vi "LEBITplc.CreateScaleAndOffsetArray.vi"(2 "DBArray":string[][](array[string]), 3 "Info Array from DB":string[][](array[string])) -> (1 "Scale And Offset Array":string[][](array[string]))   [LabVIEW 2014, in "LEBITplc.lvlib"]
uses:
  LEBITplc.lvlib
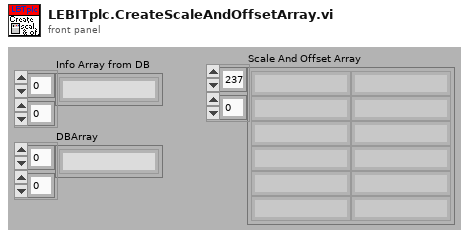
[diagram p1: front panel]
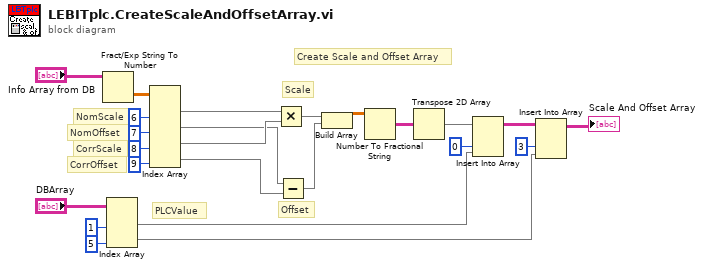
[diagram p0: block diagram]
diagram:
  # "Offset"
  # "Scale"
  # "PLCValue"
  # "Create Scale and Offset Array"
  # "CorrOffset"
  # "CorrScale"
  # "NomOffset"
  # "NomScale"
  n1 = Fract/Exp String To Number(string="Info Array from DB") -> (number=w24:dbl[][])  [unwired: 3 in, 1 out]
  n2 = Index Array(array="DBArray", index (col) #1=1 ("disabled index (col)"), index (col) #2=5 ("index (col)")) -> (element #1=w7:string[], element #2=w3:string[])  [unwired: 2 in]
  n3 = Index Array(array=w24, index (col) #1=6 ("index (col)"), index (col) #2=7 ("index (col)"), index (col) #3=8 ("index (col)"), index (col) #4=9 ("index (col)")) -> (element #1=w19:dbl[], element #2=w17:dbl[], element #3=w18:dbl[], element #4=w16:dbl[])  [unwired: 4 in]
  n4 = Multiply(x=w19, y=w18) -> (x*y=w6:dbl[])
  n5 = Subtract(x=w17, y=w16) -> (x-y=w12:dbl[])
  n6 = Build Array(w6, w12) -> (w15:dbl[][])
  n7 = Number To Fractional String(number=w15) -> (F-format string=w13:string[][])  [unwired: 3 in]
  n8 = Transpose 2D Array(2D array=w13) -> (transposed array=w9:string[][])
  n9 = Insert Into Array(array=w9, index (col)=0 ("disabled index (col)"), new element=w7) -> (w4:string[][])  [unwired: 1 in]
  n10 = Insert Into Array(array=w4, index (col)=3 ("disabled index (col)"), new element=w3) -> (→"Scale And Offset Array":string[][])  [unwired: 1 in]
